vi "SetupInterfaceLog.vi"(8 "error in (no error)":errorcluster, 11 "Model in":refnum<class "Model.lvclass">) -> (0 "error out":errorcluster, 3 "Model out":refnum<class "Model.lvclass">)   [LabVIEW 2016, in "Model.lvclass"]
uses:
  Model.lvclass
  Logging/InterfaceLogFactory.lvclass
  Model.lvclass/Model.ctl
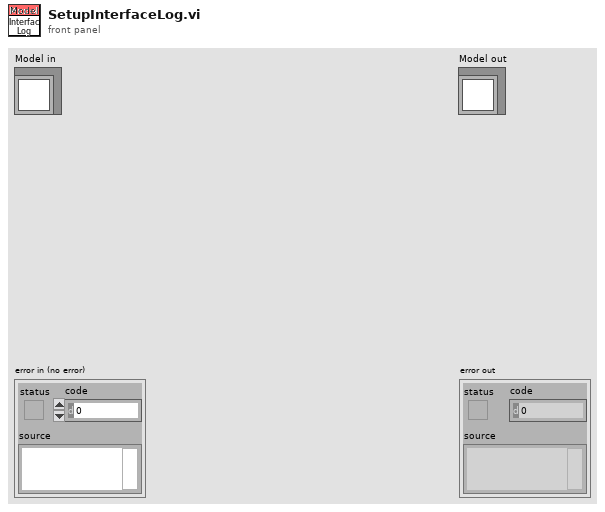
[diagram p1: front panel]
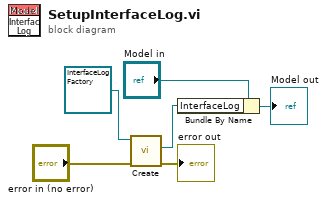
[diagram p0: block diagram]
diagram:
  n1 = call "Create.vi"("error in (no error)"="error in (no error)", "InterfaceLogFactory in"=refnum<class "InterfaceLogFactory.lvclass"> refnum ("InterfaceLogFactory.lvclass")) -> ("error out"=→"error out":errorcluster, "InterfaceLog"=w2:refnum<class "InterfaceLog.lvclass">)  [unwired: 7 in, 1 out]
  n2 = Bundle By Name(cluster="Model in", "InterfaceLog"=w2) -> (→"Model out":refnum<class "Model.lvclass">)
